vi "PLC.Dial800._TEST Read Bool Value.vi"() -> ()   [LabVIEW 2018]
panel:
  out "timestamp":timestamp
  in  "wait for updated value (T)":bool
  in  "ms timeout (1000)":i32=1000
  out "quality":u64
  out "status":u32
  out "Value":bool
  out "error out":errorcluster
  in  "URL":string="opc://localhost/RSLinx OPC Server/[Stn800]Program:Stn001_90_OffloadMain.TestPC[0].Done"
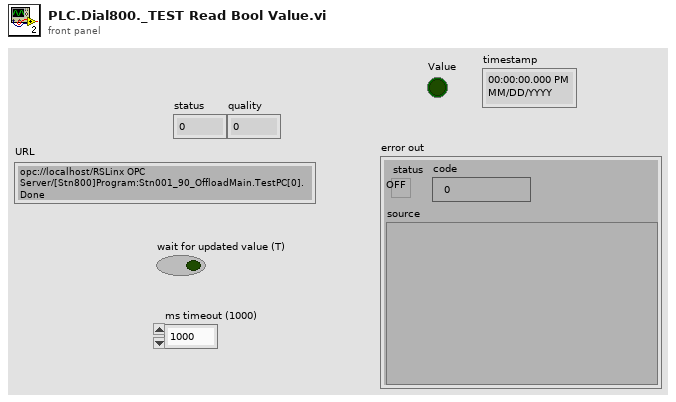
[diagram p1: front panel]
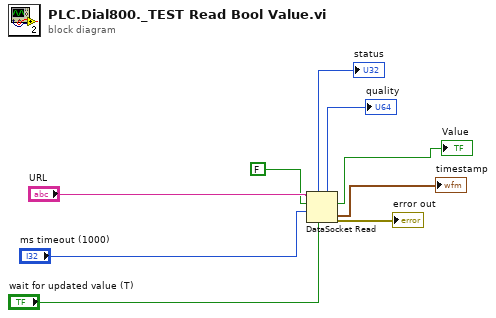
[diagram p0: block diagram]
diagram:
  n1 = DataSocket Read(6:"wait for updated value (T)", 9:"ms timeout (1000)", 10:FALSE, 11:"URL") -> (0:→"error out":errorcluster, 2:→"Value":bool, 4:→"timestamp":timestamp, 5:→"quality":u64, 7:→"status":u32)  [unwired: 1 in, 2 out]
